vi "Test register onClick event.vi"(11 "Test Case In":refnum<class "Test Cases.lvclass">) -> (0 "error out":errorcluster, 3 "Test Case Out":refnum<class "Test Cases.lvclass">)   [LabVIEW 2024, in "Test Cases.lvclass"]
uses:
  Test Cases.lvclass
  D:/git/Sourcegrid-LabVIEW/dll/SourceGrid.dll
  dll/SourceGrid.dll
  MyEventGrid/MyEventGrid.lvclass
  MyEventGrid/MyEventGrid.lvclass/MyEventGrid.ctl
  <vilib>/Astemes/LUnit/Test Case.lvclass/Test Case.ctl
  <vilib>/Astemes/LUnit/Append Pass Result.vi
  <vilib>/Astemes/LUnit/Append Fail Result.vi
  <vilib>/Astemes/LUnit/Run In UI.vi
  <vilib>/Utility/error.llb/Clear Errors.vi
  Test Cases.lvclass/Test Cases.ctl
  <vilib>/Astemes/LUnit/Test Case.lvclass
  source/Grid/SourceGrid.lvclass
panel:
  in  "Grid Container":refnum<k24>(container)
  in  "stop":bool
  out "onClick":string
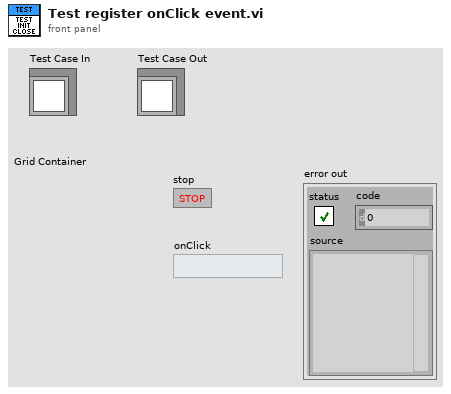
[diagram p1: front panel]
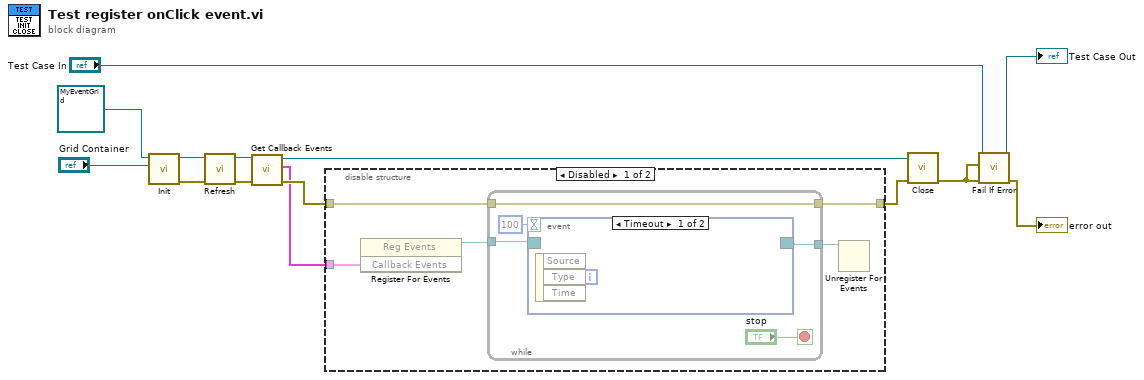
[diagram p0: block diagram]
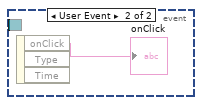
[diagram p2: hidden frame]
diagram:
  n1 = call-dynamic "Init.vi"("Sourcegrid Container"="Grid Container", "MyEventGrid in"=refnum<class "MyEventGrid.lvclass"> refnum ("Grid in")) -> ("error out"=w6:errorcluster, "MyEventGrid out"=w5:refnum<class "MyEventGrid.lvclass">)  [unwired: 8 in]
  n2 = call "Refresh.vi"("error in"=w6, "SourceGrid in"=w5) -> ("error out"=w7:errorcluster, "SourceGrid out"=w4:refnum<class "MyEventGrid.lvclass">)  [unwired: 8 in]
  n3 = call "Get Callback Events.vi"("MyEventGrid in"=w4) -> ("Callback Events"=w1:cluster{"onClick":refnum<user-event>}, "MyEventGrid out"=w3:refnum<class "MyEventGrid.lvclass">)  [unwired: 9 in]
  n4 = disable-structure shown="Disabled" {
    disable-tunnel: w7 -> [w18 w25]
    disable-tunnel: [w17 w25] -> w8
    disable-tunnel: w1 -> [w15 _]
    frame Disabled {
      n5 = register-events(w15) -> (reference out=w14:refnum<event-registration>)  [unwired: 2 in, 1 out]
      n6 = while {
        tunnel: w18 -> [w22]
        tunnel: [w22] -> w17
        tunnel: w14 -> [w21]
        tunnel: [w20] -> w16
        stop <- "stop" stop-if-true
        n7 = event shown="[0] Timeout" {
          selector: w21 -> [_ _]
          dyn-events: [_ _] -> w20
          timeout: 100 -> [_ _]
          event Timeout {
            n8 = event-data() -> ()  [unwired: 1 in, 3 out]
          }
          event User Event {
            n9 = event-data() -> ("onClick"=→"onClick":string)  [unwired: 1 in, 2 out]
          }
        }
      }
      n10 = Unregister For Events(event registration refnum=w16) -> ()  [unwired: 1 in, 1 out]
    }
    frame Enabled {
    }
  }
  n11 = call-dynamic "Close.vi"("error in"=w8, "MyEventGrid in"=w3) -> ("error out"=w2:errorcluster)  [unwired: 8 in, 1 out]
  n12 = call <vilib>:"Fail If Error.vi"("error in (no error)"=w2, "Assert error"=w2, "LUnit Test Case In"="Test Case In") -> ("error out"=→"error out":errorcluster, "LUnit Test Case Out"=→"Test Case Out":refnum<class "Test Cases.lvclass">)  [unwired: 7 in]
